vi "Write ILC.vi"(10 "ILC":refnum<class "ILC.lvclass">, 11 "ILCDAC3 in":refnum<class "ILCDAC3.lvclass">) -> (3 "ILCDAC3 out":refnum<class "ILCDAC3.lvclass">)   [LabVIEW 2015]
uses:
  ILCDAC3.lvclass
  <userlib>/Common/ILC/ILC/ILC.lvclass
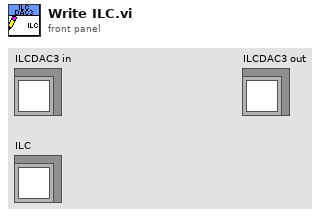
[diagram p1: front panel]
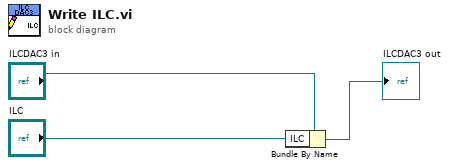
[diagram p0: block diagram]
diagram:
  n1 = Bundle By Name(cluster="ILCDAC3 in", "ILC"="ILC") -> (→"ILCDAC3 out":refnum<class "ILCDAC3.lvclass">)
